vi "CopyPattern.vi"(6 "Root":path, 8 "error in (no error)":errorcluster, 9 "SourceName":string="ROI0", 10 "CopyName":string="ROI1", 11 "SourcePatternPath":string) -> (0 "error out":errorcluster, 3 "CopyPatternPath":string)   [LabVIEW 2019]
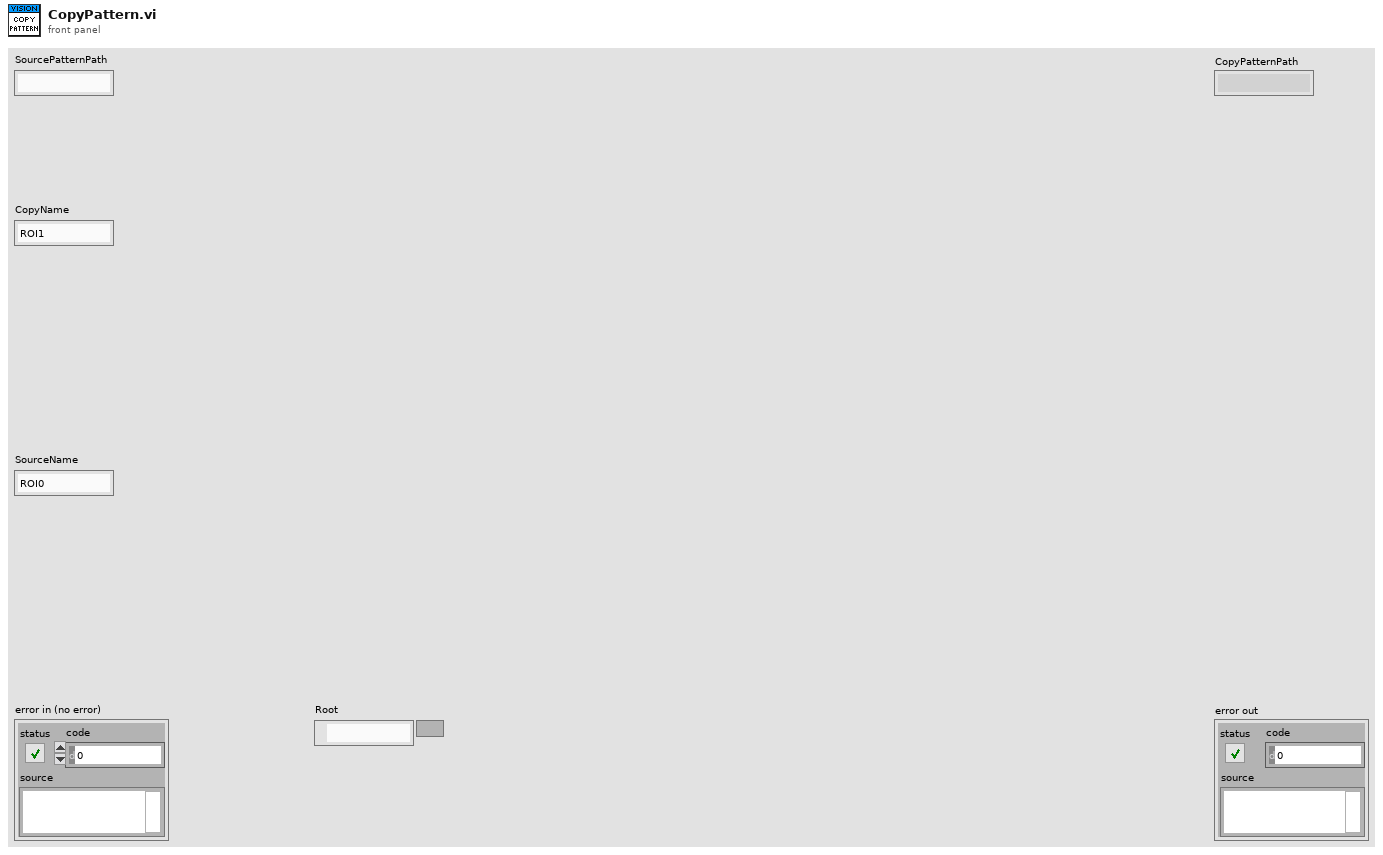
[diagram p1: front panel]
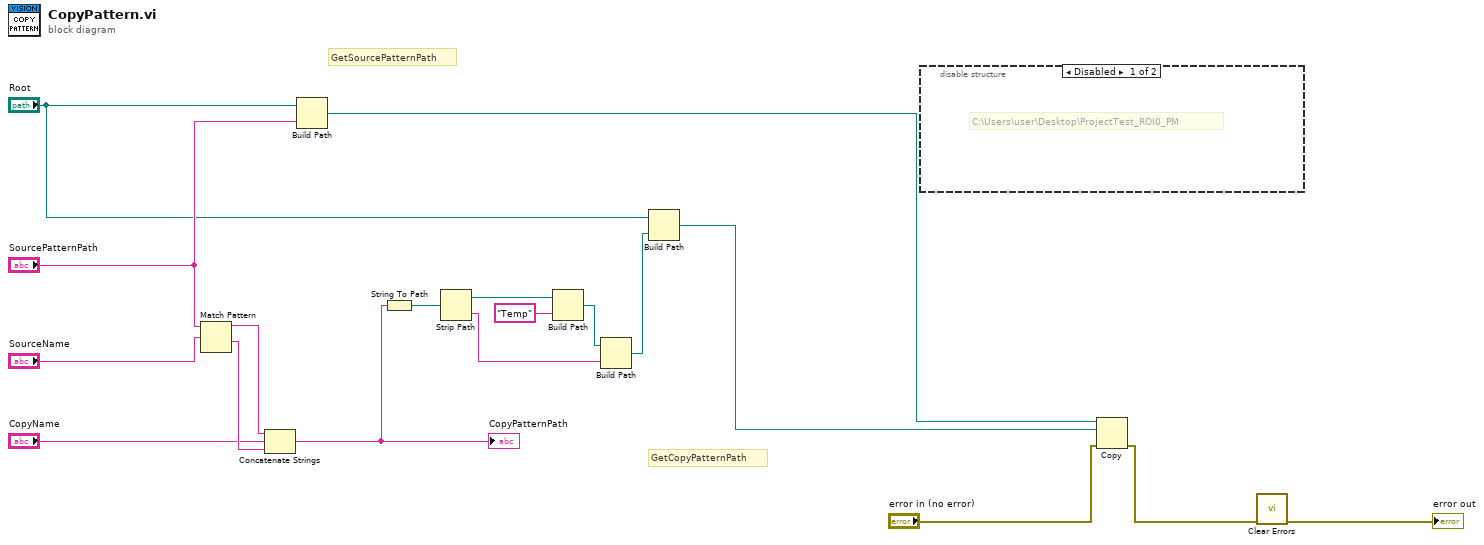
[diagram p0: block diagram]
diagram:
  # "GetCopyPatternPath"
  # "GetSourcePatternPath"
  n1 = Match Pattern(string="SourcePatternPath", regular expression="SourceName") -> (before substring=w18:string, after substring=w17:string)  [unwired: 1 in, 2 out]
  n2 = Concatenate Strings(w18, "CopyName", w17) -> (w9:string)
  "CopyPatternPath" <- w9
  n3 = Build Path(base path="Root", name or relative path="SourcePatternPath") -> (appended path=w5:path)
  n4 = String To Path(string=w9) -> (path=w13:path)
  n5 = Strip Path(path=w13) -> (stripped path=w12:path, name=w8:string)
  n6 = Build Path(base path=w12, name or relative path="Temp") -> (appended path=w10:path)
  n7 = Build Path(base path=w10, name or relative path=w8) -> (appended path=w7:path)
  n8 = Build Path(base path="Root", name or relative path=w7) -> (appended path=w4:path)
  n9 = disable-structure shown="Disabled" {
    frame Disabled {
      # "C:\\Users\\user\\Desktop\\ProjectTest_ROI0_PM"
    }
    frame Enabled {
    }
  }
  n10 = Copy(8:"error in (no error)", 10:w4, 11:w5) -> (0:w3:errorcluster)  [unwired: 2 in, 2 out]
  n11 = call <vilib>:"Clear Errors.vi"("error in (no error)"=w3) -> ("error out"=→"error out":errorcluster)  [unwired: 5 in, 1 out]
